vi "BME_DG_GetPCIDGInfo.vi"(0 "DG_Number in":i32, 11 "error in (no error)":errorcluster) -> (3 "Master":bool, 4 "DG_Number out":i32, 6 "DG_Product":i32, 8 "SlotNumber":i32, 10 "return code":i32, 15 "error out":errorcluster)   [LabVIEW 2009]
uses:
  BME DLL/DelayGenerator.dll
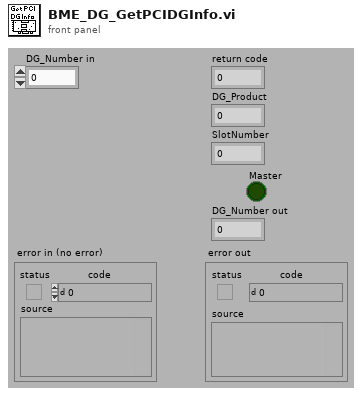
[diagram p1: front panel]
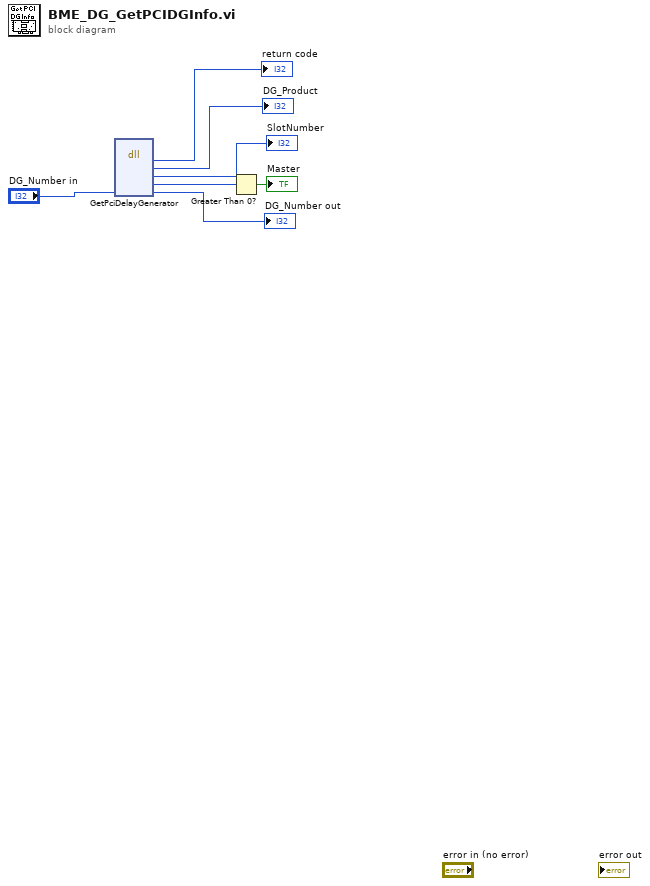
[diagram p0: block diagram]
diagram:
  n1 = dll-call lib="C:/Dokumente und Einstellungen/A2.5/Desktop/POLARIS BME DG/BME DLL/DelayGenerator.dll" fn="GetPciDelayGenerator"("DG_Number"="DG_Number in") -> (→"return code":i32, "DG_Product"=→"DG_Product":i32, "SlotNumber"=→"SlotNumber":i32, "Master"=w3:i32, "DG_Number"=→"DG_Number out":i32)  [unwired: 6 in, 2 out]
  n2 = Greater Than 0?(x=w3) -> (x > 0?=→"Master":bool)
